vi "Main_PC-Steffen’s MacBook Pro.vi"() -> ()   [LabVIEW 2018]
uses:
  <vilib>/myRIO/Instrument Drivers/Onboard IO/UART/typedef/VISA Configuration.ctl
  <vilib>/Instr/_visa.llb/VISA Configure Serial Port (Instr).vi
  <vilib>/myRIO/Instrument Drivers/Onboard IO/UART/UART.lvlib
panel:
  out "Drilling Process":string
  out "RollDetection":bool
  out "Ready to Fly":bool
  in  "stop":bool
  out "error out":errorcluster
  in  "error in (no error)":errorcluster
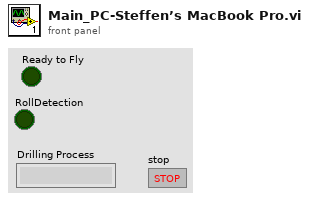
[diagram p1: front panel]
types:
  T1 = typedef "UART.lvlib/VISA Configuration.ctl" = cluster{"baud rate (9600)":u32, "data bits (8)":u16, "parity (0:none)":enum16{"None", "Odd", "Even", "Mark", "Space"}, "stop bits (10: 1 bit)":u16, "flow control (0:none)":u16, "termination char\n(0xA = '\\n' = LF) ":u8, "Enable Termination\nChar (T)":bool, "timeout (10sec)":u32}
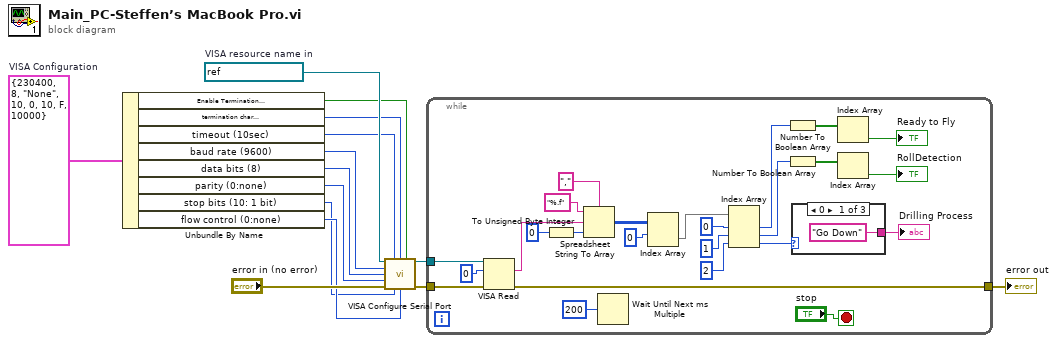
[diagram p0: block diagram]
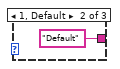
[diagram p2: hidden frame]
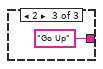
[diagram p3: hidden frame]
diagram:
  w13 = T1 {"baud rate (9600)"=230400, "data bits (8)"=8, "parity (0:none)"=enum."None", "stop bits (10: 1 bit)"=10, "flow control (0:none)"=0, "termination char\n(0xA = '\\n' = LF) "=10, "Enable Termination\nChar (T)"=FALSE, "timeout (10sec)"=10000}  # VISA Configuration
  w14 = refnum<visa-resource-name> "ASRL2::INSTR"  # VISA resource name in
  n1 = Unbundle By Name(w13) -> ("Enable Termination\nChar (T)"=w9:bool, "termination char\n(0xA = '\\n' = LF)"=w8:u8, "timeout (10sec)"=w7:u32, "baud rate (9600)"=w2:u32, "data bits (8)"=w3:u16, "parity (0:none)"=w4:enum16{"None", "Odd", "Even", "Mark", "Space"}, "stop bits (10: 1 bit)"=w5:u16, "flow control (0:none)"=w6:u16)
  n2 = call-poly "VISA Configure Serial Port"("VISA resource name"=w14, "timeout (10sec)"=w7, "termination char\n(0xA = '\\n' = LF)"=w8, "Enable Termination\nChar (T)"=w9, "baud rate (9600)"=w2, "data bits (8)"=w3, "parity (0:none)"=w4, "error in (no error)"="error in (no error)", "stop bits (10: 1 bit)"=w5, "flow control (0:none)"=w6) -> ("VISA resource name out"=w11:refnum<visa-resource-name>, "error out"=w10:errorcluster)  [unwired: 4 in]
  n3 = while {
    tunnel: w11 -> [w37]
    tunnel: w10 -> [w36]
    tunnel: [w35] -> w1
    stop <- "stop" stop-if-true
    n4 = VISA Read(VISA resource name=w37, byte count=u32 0 ("Character Count"), error in (no error)=w36) -> (read buffer=w33:string, error out=w35:errorcluster)  [unwired: 2 out]
    n5 = To Unsigned Byte Integer(number=0) -> (unsigned 8bit integer=w30:u8)
    n6 = Spreadsheet String To Array(delimiter (Tab)=",", format string="%.f", spreadsheet string=w33, array type (2D Dbl)=w30) -> (array=w27:u8[][])
    n7 = Wait Until Next ms Multiple(millisecond multiple=u32 200) -> ()  [unwired: 1 out]
    n8 = Index Array(array=w27, index (row)=0) -> (element=w25:u8[])  [unwired: 1 in]
    n9 = Index Array(array=w25, index #1=0 ("index (row)"), index #2=1 ("index"), index #3=2 ("index")) -> (element #1=w22:u8, element #2=w18:u8, element #3=w16:u8)
    n10 = Number To Boolean Array(number=w22) -> (Boolean array=w21:bool[])
    n11 = Number To Boolean Array(number=w18) -> (Boolean array=w19:bool[])
    n12 = case shown="0" w16 {
      tunnel: ["Go Down" "Default" "Go Up"] -> w15
      frame 0 {
      }
      frame 1, Default {
      }
      frame 2 {
      }
    }
    "Drilling Process" <- w15
    n13 = Index Array(array=w21) -> (element=→"Ready to Fly":bool)  [unwired: 1 in]
    n14 = Index Array(array=w19) -> (element=→"RollDetection":bool)  [unwired: 1 in]
  }
  "error out" <- w1
